vi "AverageOneCoordOld(SubVI).vi"(0 "Array":dbl[](array[numeric]), 9 "Number of pins":i32=5, 11 "Number of images each":i32=10) -> (4 "Top Averages":dbl[][](array[numeric]), 6 "Bottom averages":dbl[][](array[numeric]), 8 "Top SD":dbl[][](array[numeric]), 10 "Bottom SD":dbl[][](array[numeric]))   [LabVIEW 2016]
uses:
  <vilib>/Analysis/NI_AALBase.lvlib
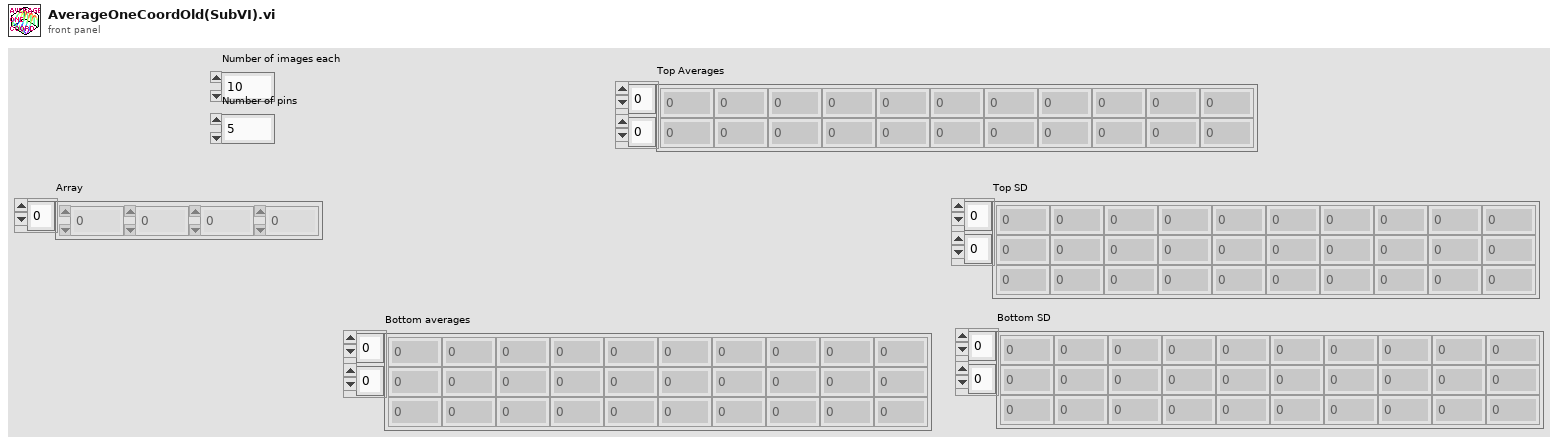
[diagram p1: front panel]
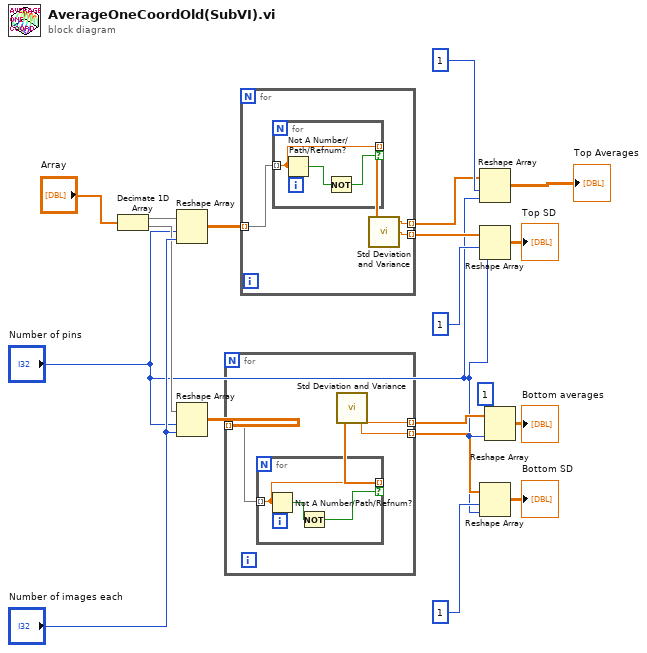
[diagram p0: block diagram]
diagram:
  n1 = Decimate 1D Array("Array") -> (w18:dbl[], w3:dbl[])
  n2 = Reshape Array(w18, "Number of pins", "Number of images each") -> (w17:dbl[][])
  n3 = Reshape Array(w3, "Number of pins", "Number of images each") -> (w16:dbl[][])
  n4 = for {
    tunnel: w16 -> [w21] mode=indexing
    tunnel: [w23] -> w5 mode=indexing
    tunnel: [w22] -> w4 mode=indexing
    n5 = for {
      tunnel: w21 -> [w26] mode=indexing
      tunnel: [w26] -> w20 mode=indexing if=w24
      n6 = Not A Number/Path/Refnum?(number/path/refnum=w26) -> (NaN/Path/Refnum?=w25:bool)
      n7 = Not(x=w25) -> (.not. x?=w24:bool)
    }
    n8 = call <vilib>:"Std Deviation and Variance.vi"("X"=w20) -> ("mean"=w23:dbl, "standard deviation"=w22:dbl)  [unwired: 1 in, 1 out]
  }
  n9 = for {
    tunnel: w17 -> [w28] mode=indexing
    tunnel: [w30] -> w7 mode=indexing
    tunnel: [w29] -> w6 mode=indexing
    n10 = for {
      tunnel: w28 -> [w33] mode=indexing
      tunnel: [w33] -> w27 mode=indexing if=w31
      n11 = Not A Number/Path/Refnum?(number/path/refnum=w33) -> (NaN/Path/Refnum?=w32:bool)
      n12 = Not(x=w32) -> (.not. x?=w31:bool)
    }
    n13 = call <vilib>:"Std Deviation and Variance.vi"("X"=w27) -> ("mean"=w30:dbl, "standard deviation"=w29:dbl)  [unwired: 1 in, 1 out]
  }
  n14 = Reshape Array(w7, 1 ("dimension size"), "Number of pins") -> (→"Top Averages":dbl[][])
  n15 = Reshape Array(w6, 1 ("dimension size"), "Number of pins") -> (→"Top SD":dbl[][])
  n16 = Reshape Array(w4, 1 ("dimension size"), "Number of pins") -> (→"Bottom SD":dbl[][])
  n17 = Reshape Array(w5, 1 ("dimension size"), "Number of pins") -> (→"Bottom averages":dbl[][])
